vi "Laurel Modbus Example.vi"() -> ()   [LabVIEW 2019]
uses:
  <vilib>/NI/Modbus Library/API/Wrapper/Create TCP Master.vi
  <vilib>/NI/Modbus Library/API/Master/Modbus Master.lvclass
  <vilib>/NI/Modbus Library/API/Wrapper/API Main.lvlib
panel:
  in  "Reset Total":bool
  out "Rate Only":dbl
  out "Rate":dbl
  out "Totalizer":dbl
  out "Error Out":errorcluster
  in  "Remote IP Address":string="10.2.0.14"
  in  "Error In":errorcluster
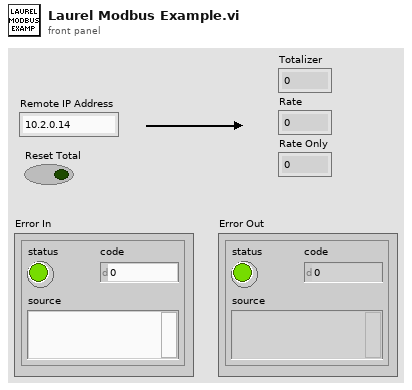
[diagram p1: front panel]
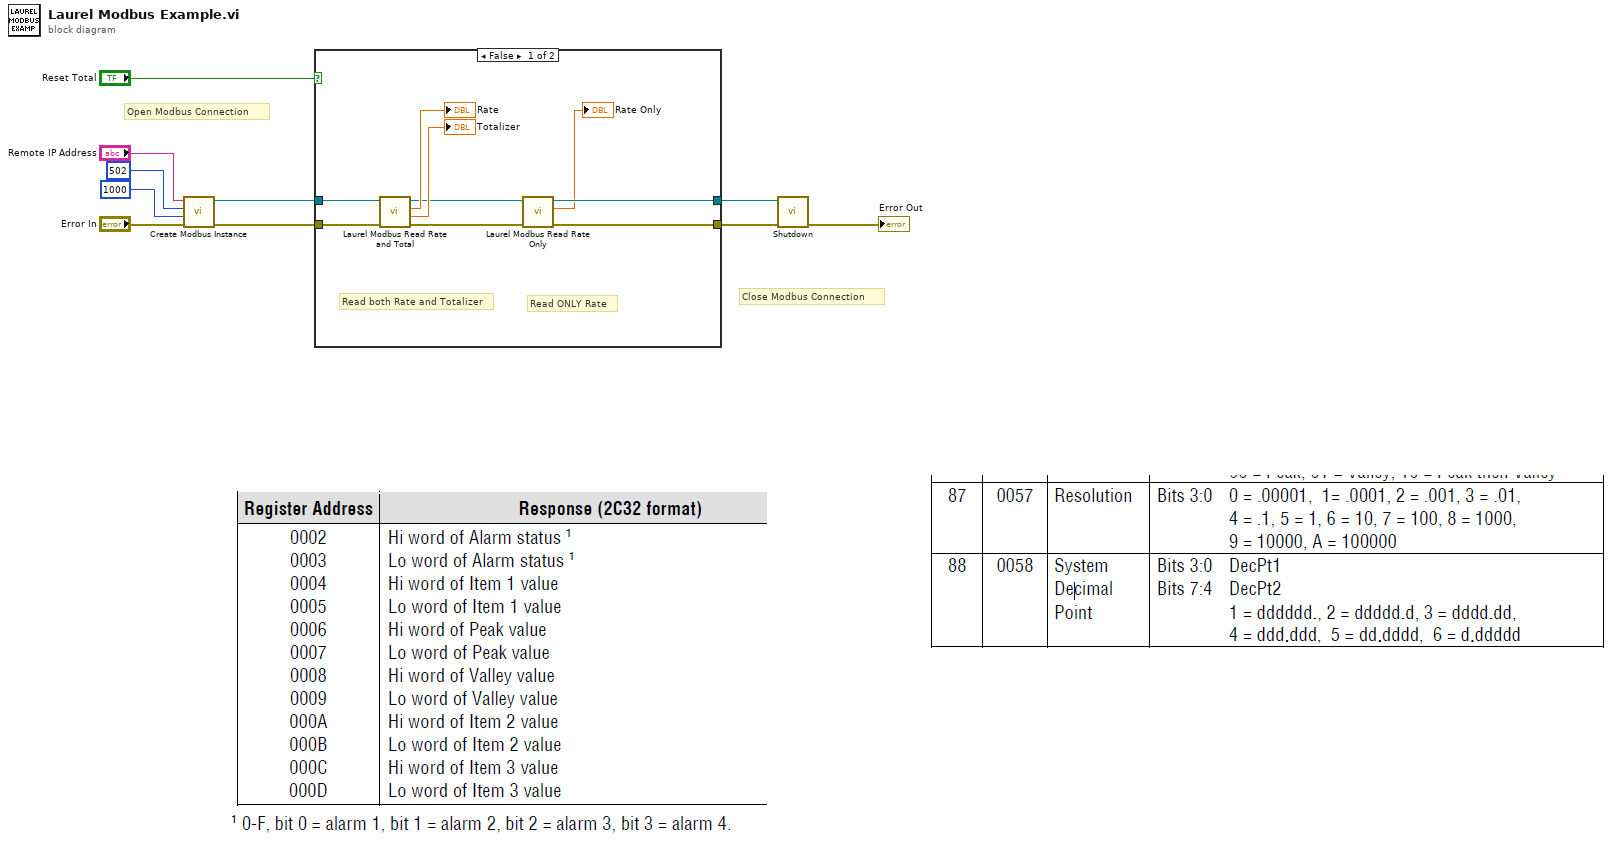
[diagram p0: block diagram]
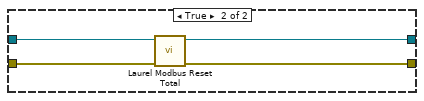
[diagram p2: hidden frame]
diagram:
  # "Close Modbus Connection"
  # "Open Modbus Connection"
  n1 = call-poly <vilib>:"Create Modbus Instance.vi"("error in"="Error In", "connect timeout ms"=1000, "port (502)"=u16 502, "address"="Remote IP Address") -> ("error out"=w4:errorcluster, "TCP master instance"=w5:refnum<class "Modbus Master.lvclass">)  [unwired: 6 in]
  n2 = case shown="False" "Reset Total" {
    tunnel: w5 -> [w19 w23]
    tunnel: w4 -> [w18 w22]
    tunnel: [w13 w21] -> w3
    tunnel: [w12 w20] -> w2
    frame False {
      # "Read ONLY Rate"
      # "Read both Rate and Totalizer"
      n3 = call "Laurel Modbus Read Rate and Total.vi"("error in (no error)"=w18, "Modbus Master in"=w19) -> ("error out"=w14:errorcluster, "Totalizer"=→"Totalizer":dbl, "Rate"=→"Rate":dbl, "Modbus Master out"=w15:refnum<class "Modbus Master.lvclass">)  [unwired: 6 in]
      n4 = call "Laurel Modbus Read Rate Only.vi"("error in (no error)"=w14, "Modbus Master in"=w15) -> ("error out"=w12:errorcluster, "Rate"=→"Rate Only":dbl, "Modbus Master out"=w13:refnum<class "Modbus Master.lvclass">)  [unwired: 7 in]
    }
    frame True {
      n5 = call "Laurel Modbus Reset Total.vi"("Error In"=w22, "Modbus Master in"=w23) -> ("Error Out"=w20:errorcluster, "Modbus Master out"=w21:refnum<class "Modbus Master.lvclass">)  [unwired: 8 in]
    }
  }
  n6 = call-dynamic "Shutdown.vi"("error in"=w2, "Modbus master in"=w3) -> ("error out"=→"Error Out":errorcluster)  [unwired: 9 in]
